vi "Example-SimpleTranslator.vi"() -> ()   [LabVIEW 2015]
uses:
  lvlib/TargetLang.ctl
  lvlib/Translate_Standard.vi
  lvlib/lv-deepl-api.lvlib
panel:
  in  "TargetLang":T1
  in  "API key":string
  in  "Translate":bool
  out "Translate Result":string
  in  "Input Text":string
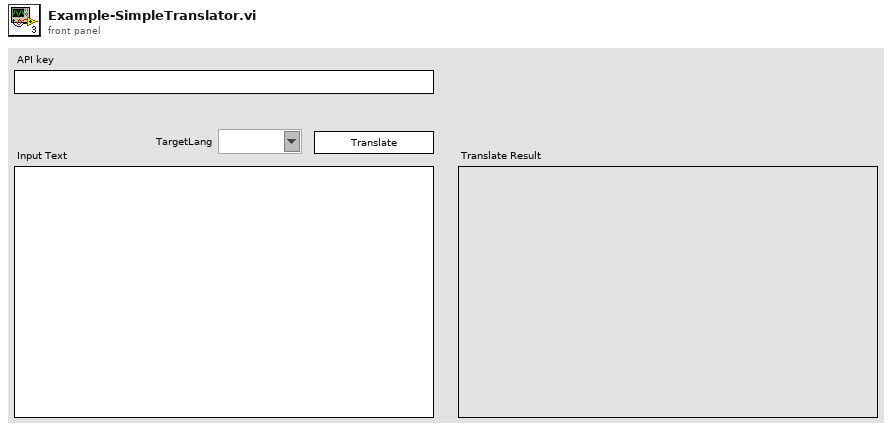
[diagram p1: front panel]
types:
  T1 = typedef "lv-deepl-api.lvlib/TargetLang.ctl" = string
  T2 = cluster{"detected_source_language":string, "text":string}[]
  T3 = cluster{"detected_source_language":string, "text":string}
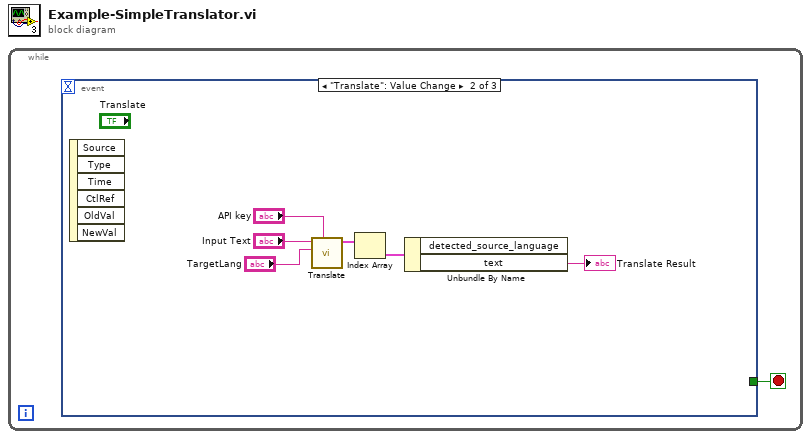
[diagram p0: block diagram]
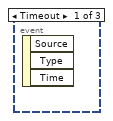
[diagram p2: hidden frame]
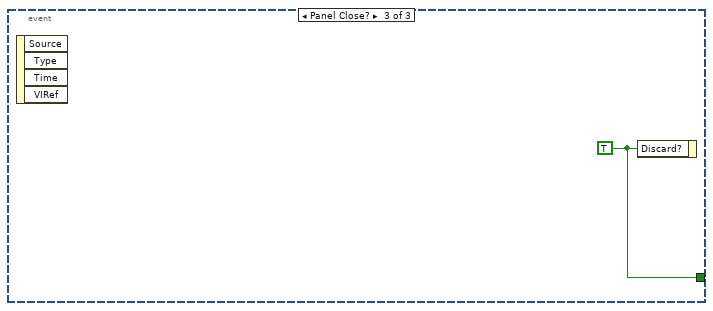
[diagram p3: hidden frame]
diagram:
  n1 = while {
    stop <- w1 stop-if-true
    n2 = event shown="[1] \"Translate\": Value Change" {
      selector: _ -> [_ _ _]
      dyn-events: _ -> [_ _ _]
      timeout: _ -> [_ _ _]
      tunnel: [_ _ w8] -> w1
      event Timeout {
        n3 = event-data() -> ()  [unwired: 1 in, 3 out]
      }
      event "Translate": Value Change {
        n4 = event-data() -> ()  [unwired: 1 in, 6 out]
        n5 = call-poly "Translate.vi"("DeepL authKey"="API key", "TargetLang"="TargetLang", "Input text"="Input Text") -> ("translations"=w6:T2)  [unwired: 7 in, 1 out]
        n6 = Index Array(array=w6) -> (element=w5:T3)  [unwired: 1 in]
        n7 = Unbundle By Name(w5) -> ("text"=→"Translate Result":string)  [unwired: 1 out]
      }
      event Panel Close? {
        w8 = TRUE ("Discard?")
        n8 = event-data() -> ()  [unwired: 1 in, 4 out]
        n9 = event-data("Discard?"=w8) -> ()  [unwired: 1 in, 1 out]
      }
    }
  }
